vi "Get Frame Time Info.vi"(8 "Frame Index":i32, 9 "Current Time Stamp":timestamp, 10 "Settings.Incoming Values":T1) -> (2 "Settings.Incoming Values out":T1)   [LabVIEW 2019, in "Protection and Counter Support Engine.lvlib"]
uses:
  Types/RT Frame Incoming Values.ctl
  Protection and Counter Support Engine.lvlib
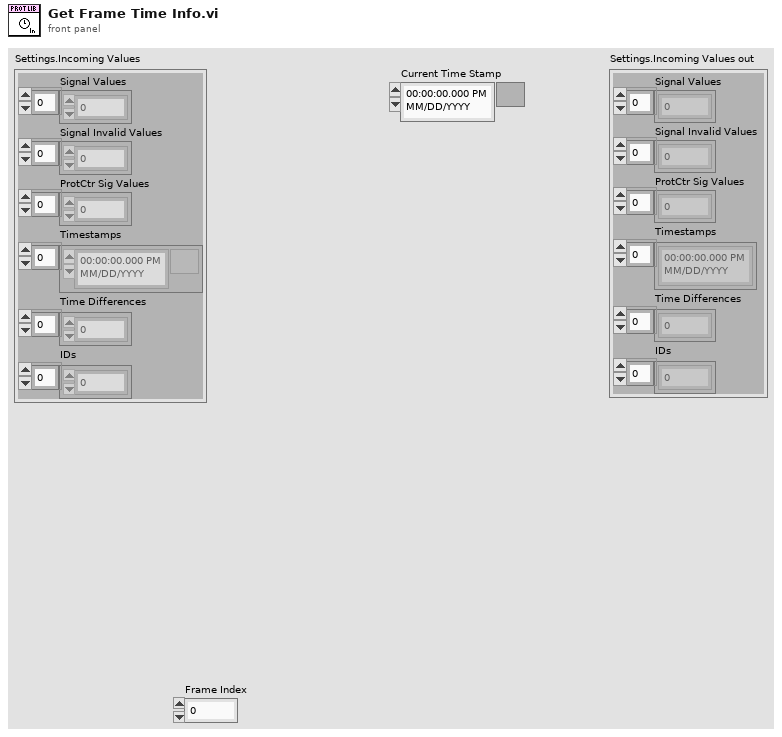
[diagram p1: front panel]
types:
  T1 = typedef "Protection and Counter Support Engine.lvlib/RT Frame Incoming Values.ctl" = cluster{"Signal Values":dbl[], "Signal Invalid Values":dbl[], "ProtCtr Sig Values":dbl[], "Timestamps":timestamp[], "Time Differences":dbl[], "IDs":u32[]}
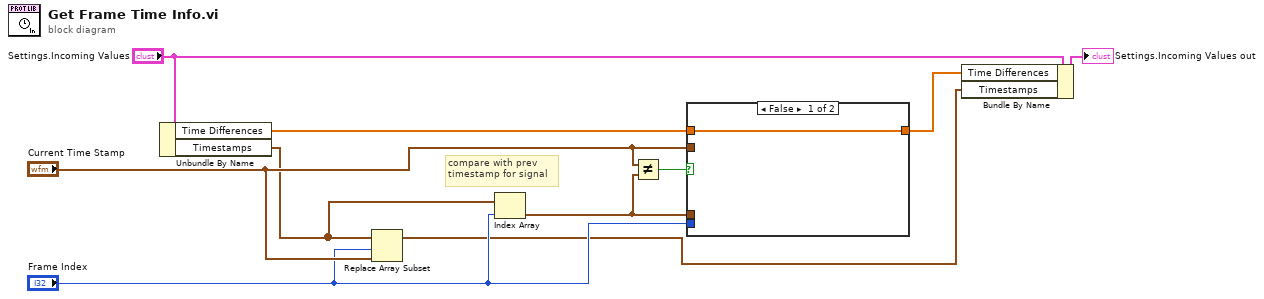
[diagram p0: block diagram]
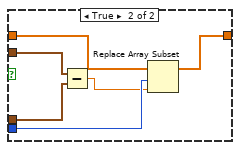
[diagram p2: hidden frame]
diagram:
  # "compare with prev\ntimestamp for signal"
  n1 = Unbundle By Name("Settings.Incoming Values") -> ("Time Differences"=w5:dbl[], "Timestamps"=w4:timestamp[])
  n2 = Replace Array Subset(array=w4, new element="Current Time Stamp", index="Frame Index") -> (w1:timestamp[])
  n3 = Index Array(array=w4, index="Frame Index") -> (element=w10:timestamp)
  n4 = Not Equal?(x="Current Time Stamp", y=w10) -> (x != y?=w9:bool)
  n5 = case shown="False" w9 {
    tunnel: "Current Time Stamp" -> [_ w17]
    tunnel: w10 -> [_ w16]
    tunnel: "Frame Index" -> [_ w15]
    tunnel: w5 -> [w11 w13]
    tunnel: [w11 w12] -> w2
    frame False {
    }
    frame True {
      n6 = Subtract(x=w17, y=w16) -> (x-y=w14:dbl)
      n7 = Replace Array Subset(array=w13, new element=w14, index=w15) -> (w12:dbl[])
    }
  }
  n8 = Bundle By Name(cluster="Settings.Incoming Values", "Time Differences"=w2, "Timestamps"=w1) -> (→"Settings.Incoming Values out":T1)
